vi "paraCfgEditor.vi"() -> ()   [LabVIEW 2010]
panel:
  in  "para section":string(tree)="parameter section"
  in  "Parameter CFG EDIT":string[][](table)
  out "View row details":string[](array[string])
  out "error out":errorcluster
  in  "error in":errorcluster
  in  "stop":bool
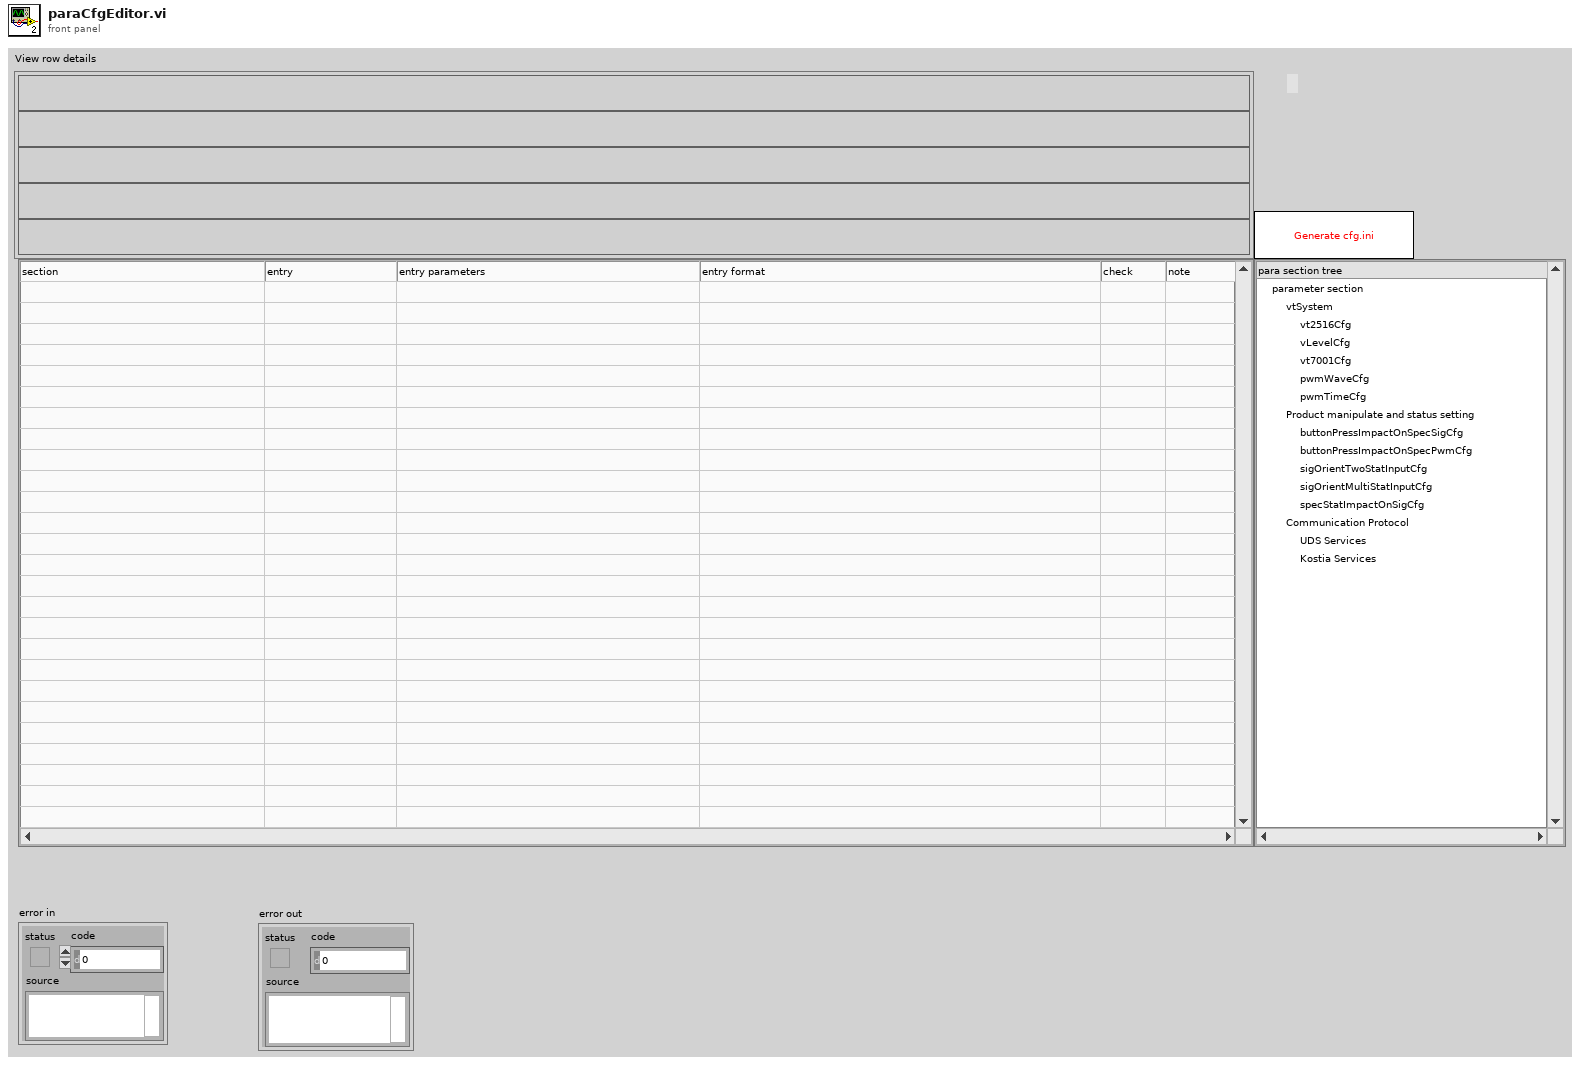
[diagram p1: front panel]
types:
  T1 = typedef "LVRowAndColumnTypeDef.ctl" = cluster{"Row":i32, "Column":i32}
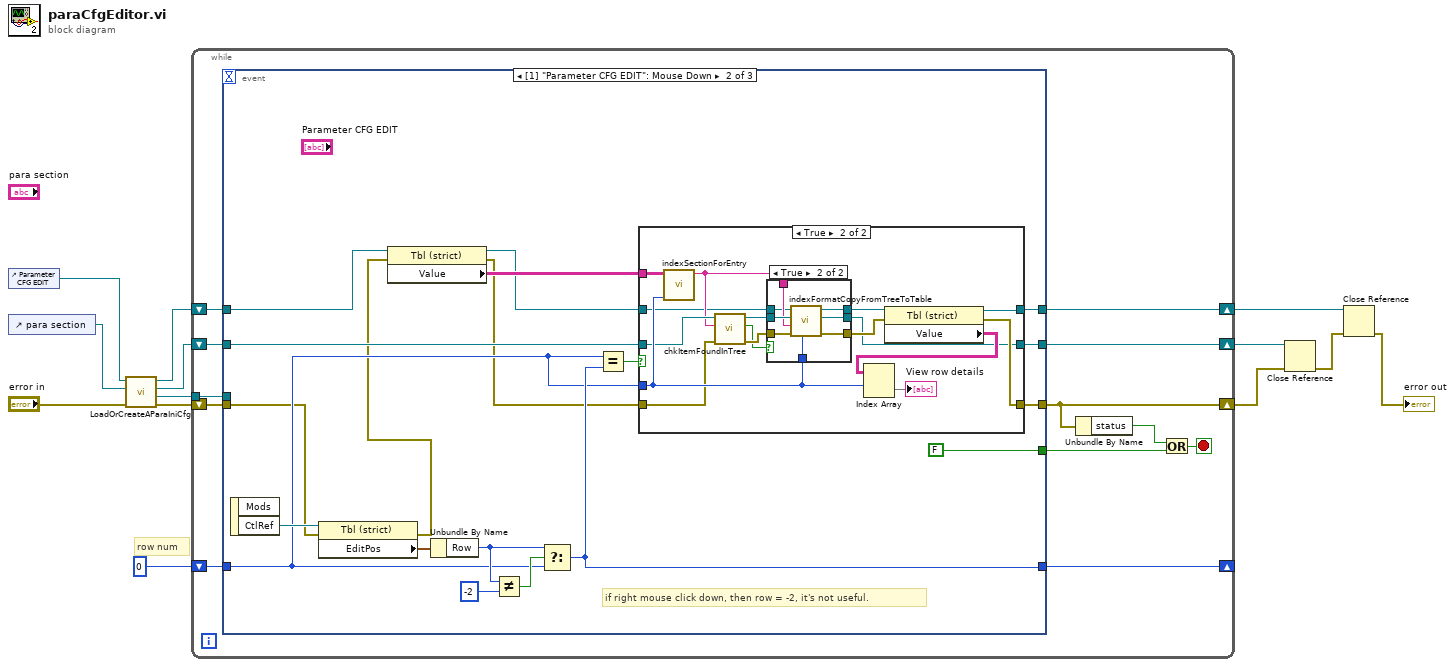
[diagram p0: block diagram]
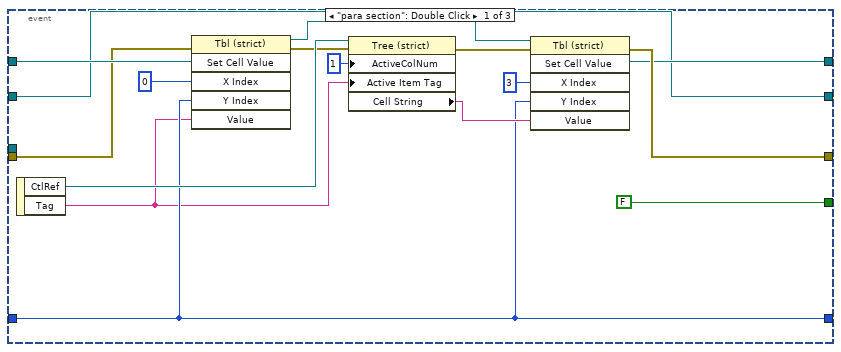
[diagram p2: hidden frame]
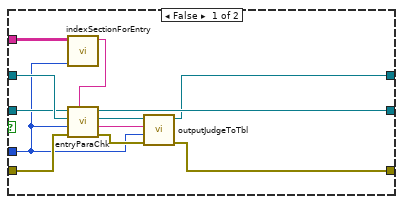
[diagram p3: hidden frame]
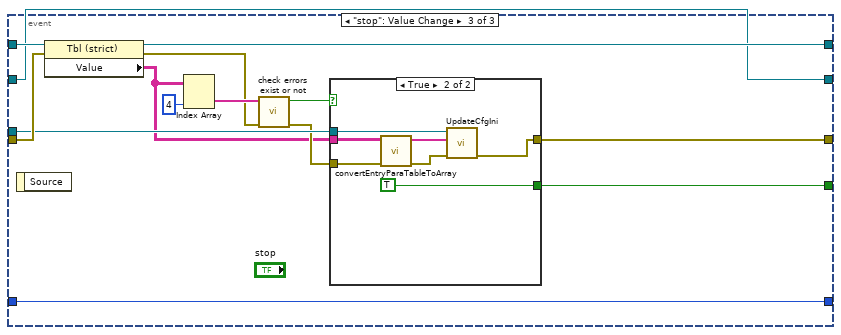
[diagram p5: hidden frame]
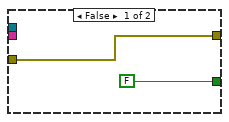
[diagram p6: hidden frame]
diagram:
  # "row num"
  n1 = control-ref of="Parameter CFG EDIT"() -> (w2:refnum<vi>)
  n2 = control-ref of="para section"() -> (w1:refnum<vi>)
  n3 = call "LoadOrCreateAParaIniCfg.vi"("error in"="error in", "Tree Refnum"=w1, "Tbl Refnum in"=w2) -> ("error out"=w8:errorcluster, "cfg file refnum out"=w12:refnum<file>, "Tree Refnum out"=w7:refnum<vi>, "Tbl Refnum out"=w9:refnum<vi>)  [unwired: 5 in]
  n4 = while {
    shift-right: [w22] -> w5
    shift-left: w8 -> [w25]
    shift-right: [w18] -> _
    shift-left: 0 ("Row") -> [w19]
    shift-right: [w17] -> w11
    shift-left: w9 -> [w20]
    tunnel: w12 -> [w16]
    shift-right: [w14] -> w6
    shift-left: w7 -> [w15]
    stop <- w23 stop-if-true
    n5 = event shown="[1] \"Parameter CFG EDIT\": Mouse Down" {
      selector: _ -> [_ _ _]
      dyn-events: _ -> [_ _ _]
      timeout: _ -> [_ _ _]
      tunnel: w25 -> [w40 w49 w109]
      tunnel: [w31 w55 w110] -> w22
      tunnel: [FALSE ("stop") FALSE ("stop") w113] -> w24
      tunnel: w20 -> [w41 w46 w111]
      tunnel: w19 -> [w29 w51 w112]
      tunnel: [w29 w53 w112] -> w18
      tunnel: [w28 w52 w104] -> w17
      tunnel: w16 -> [_ _ w108]
      tunnel: w15 -> [w27 w48 w100]
      tunnel: [w27 w47 w100] -> w14
      event "para section": Double Click {
        n6 = event-data() -> ("CtlRef"=w38:refnum<vi>, "Tag"=w26:string)  [unwired: 1 in]
        n7 = invoke class="Tbl (strict)" method="Set Cell Value"(reference=w41, error in=w40, "X Index"=u32 0 ("Y Index"), "Y Index"=w29, "Value"=w26) -> (reference out=w32:refnum<vi>, error out=w33:errorcluster)  [unwired: 1 in, 4 out]
        n8 = property class="Tree (strict)"(reference=w38, error in=w33, "ActiveColNum"=1 ("Active Cell:Active Column Number"), "Active Item Tag"=w26) -> (error out=w36:errorcluster, "Cell String"=w35:string)  [unwired: 1 out]
        n9 = invoke class="Tbl (strict)" method="Set Cell Value"(reference=w32, error in=w36, "X Index"=u32 3, "Y Index"=w29, "Value"=w35) -> (reference out=w28:refnum<vi>, error out=w31:errorcluster)  [unwired: 1 in, 4 out]
      }
      event "Parameter CFG EDIT": Mouse Down {
        # "if right mouse click down, then row = -2, it's not useful."
        n10 = event-data() -> ("CtlRef"=w60:refnum<vi>)  [unwired: 1 in, 1 out]
        n11 = property class="Tbl (strict)"(reference=w60, error in=w49) -> (error out=w45:errorcluster, "EditPos"=w59:T1)  [unwired: 1 out]
        n12 = property class="Tbl (strict)"(reference=w46, error in=w45) -> (reference out=w42:refnum<vi>, error out=w43:errorcluster, "Value"=w44:string[][])
        n13 = Unbundle By Name(w59) -> ("Row"=w56:i32)
        n14 = Not Equal?(x=w56, y=-2) -> (x != y?=w57:bool)
        n15 = Select(t=w56, s=w57, f=w51) -> (s? t:f=w53:i32)
        n16 = Equal?(x=w51, y=w53) -> (x = y?=w54:bool)
        n17 = case shown="True" w54 {
          tunnel: w51 -> [w63 w82]
          tunnel: w42 -> [w71 w73]
          tunnel: w43 -> [w72 w77]
          tunnel: [w64 w81] -> w55
          tunnel: [w65 w84] -> w52
          tunnel: w48 -> [w70 w79]
          tunnel: [w69 w80] -> w47
          tunnel: w44 -> [w62 w87]
          frame False {
            n18 = call "indexSectionForEntry.vi"("rowNum"=w63, "tbl"=w62) -> ("indexSection"=w61:string)  [unwired: 9 in]
            n19 = call "entryParaChk.vi"("indexSec"=w61, "error in"=w72, "Row number"=w63, "Tbl Refnum in"=w71, "Tree Refnum in"=w70) -> ("error out"=w67:errorcluster, "Check result"=w68:string, "Tbl Refnum out"=w66:refnum<vi>, "Tree Refnum out"=w69:refnum<vi>)  [unwired: 3 in]
            n20 = call "outputJudgeToTbl.vi"("error in"=w67, "rowNum"=w63, "judgeRes"=w68, "Tbl Refnum in"=w66) -> ("error out"=w64:errorcluster, "Tbl Refnum Out"=w65:refnum<vi>)  [unwired: 6 in]
          }
          frame True {
            n21 = call "indexSectionForEntry.vi"("rowNum"=w82, "tbl"=w87) -> ("indexSection"=w75:string)  [unwired: 9 in]
            n22 = call "chkItemFoundInTree.vi"("error in"=w77, "searchItem"=w75, "Tree Refnum in"=w79) -> ("error out"=w76:errorcluster, "FoundInTree?"=w74:bool, "Tree Refnum out"=w78:refnum<vi>)  [unwired: 6 in]
            n23 = case shown="True" w74 {
              tunnel: [w91 w99] -> w86
              tunnel: [w89 w98] -> w85
              tunnel: w82 -> [_ w97]
              tunnel: [w90 w96] -> w80
              tunnel: w78 -> [w90 w95]
              tunnel: w76 -> [w89 w94]
              tunnel: w75 -> [_ w93]
              tunnel: w73 -> [w91 w92]
              frame False {
              }
              frame True {
                n24 = call "indexFormatCopyFromTreeToTable.vi"("rowNum"=w97, "error in"=w94, "searchItem"=w93, "Tree Refnum In"=w95, "Tbl Refnum in"=w92) -> ("error out"=w98:errorcluster, "Tree Refnum Out"=w96:refnum<vi>, "Tbl Refnum Out"=w99:refnum<vi>)  [unwired: 4 in]
              }
            }
            n25 = property class="Tbl (strict)"(reference=w86, error in=w85) -> (reference out=w84:refnum<vi>, error out=w81:errorcluster, "Value"=w83:string[][])
            n26 = Index Array(array=w83, index (row)=w82) -> (element=→"View row details":string[])  [unwired: 1 in]
          }
        }
      }
      event "stop": Value Change {
        n27 = event-data() -> ()  [unwired: 1 in, 1 out]
        n28 = property class="Tbl (strict)"(reference=w111, error in=w109) -> (reference out=w104:refnum<vi>, error out=w105:errorcluster, "Value"=w101:string[][])
        n29 = Index Array(array=w101, index (col)=4 ("disabled index (col)")) -> (element=w106:string[])  [unwired: 1 in]
        n30 = call "check errors exist or not.vi"("error in"=w105, "judge column"=w106) -> ("error out"=w103:errorcluster, "Go on?"=w102:bool)  [unwired: 8 in]
        n31 = case shown="True" w102 {
          tunnel: [FALSE ("stop") TRUE ("stop")] -> w113
          tunnel: [w114 w121] -> w110
          tunnel: w108 -> [_ w116]
          tunnel: w103 -> [w114 w120]
          tunnel: w101 -> [_ w119]
          frame False {
          }
          frame True {
            n32 = call "convertEntryParaTableToArray.vi"("error in"=w120, "entryParaTbl"=w119) -> ("error out"=w118:errorcluster, "contArr"=w117:string[])  [unwired: 8 in]
            n33 = call "UpdateCfgIni.vi"("error in"=w118, "contentArray"=w117, "iniCfgRefnumIn"=w116) -> ("error out"=w121:errorcluster)  [unwired: 8 in]
          }
        }
      }
    }
    n34 = Unbundle By Name(w22) -> ("status"=w21:bool)
    n35 = Or(x=w21, y=w24) -> (x .or. y?=w23:bool)
  }
  n36 = Close Reference(reference=w6, error in (no error)=w5) -> (error out=w4:errorcluster)
  n37 = Close Reference(reference=w11, error in (no error)=w4) -> (error out=→"error out":errorcluster)
